vi "A01423754_Ximena_Avila_Ejercicio_16_examen_11_Febrero.vi"() -> ()   [LabVIEW 2018]
panel:
  in  "stop":bool
  out "a":bool
  out "b":bool
  out "c":bool
  out "d":bool
  out "e":bool
  out "f":bool
  out "g":bool
  out "7":bool
  out "6":bool
  out "4":bool
  out "5":bool
  out "3":bool
  out "2":bool
  out "1":bool
  in  "Boolean7":bool
  in  "Boolean6":bool
  in  "Boolean5":bool
  in  "Boolean4":bool
  in  "Boolean3":bool
  in  "Boolean2":bool
  in  "Boolean1":bool
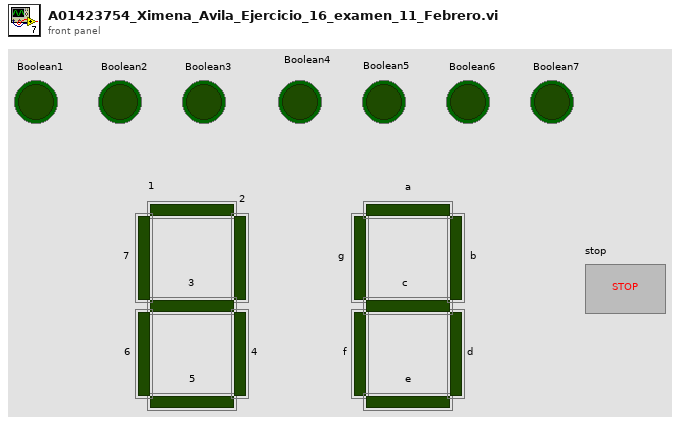
[diagram p1: front panel]
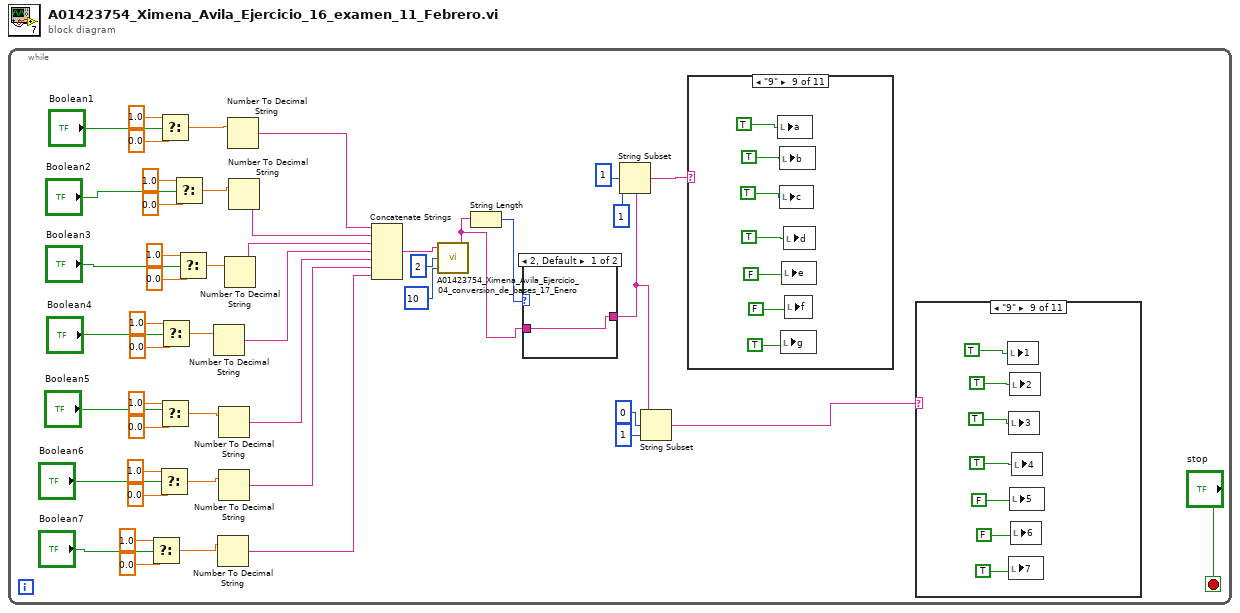
[diagram p0: block diagram]
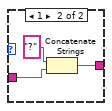
[diagram p2: hidden frame]
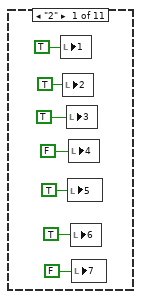
[diagram p3: hidden frame]
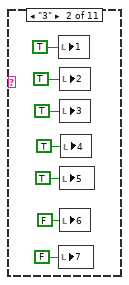
[diagram p4: hidden frame]
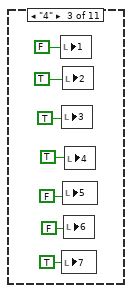
[diagram p5: hidden frame]
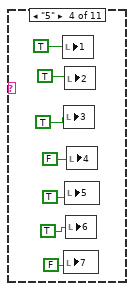
[diagram p6: hidden frame]
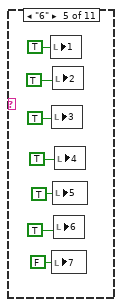
[diagram p7: hidden frame]
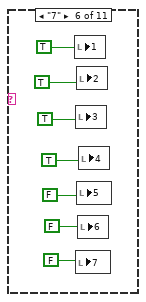
[diagram p8: hidden frame]
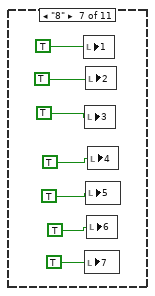
[diagram p9: hidden frame]
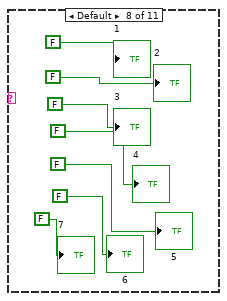
[diagram p10: hidden frame]
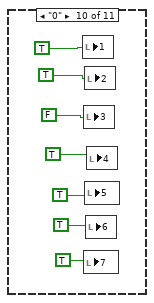
[diagram p11: hidden frame]
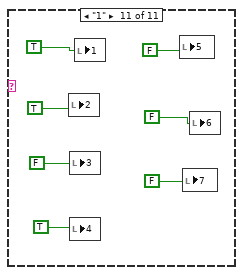
[diagram p12: hidden frame]
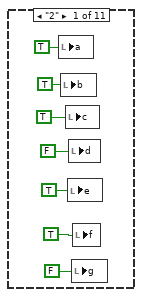
[diagram p13: hidden frame]
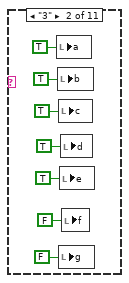
[diagram p14: hidden frame]
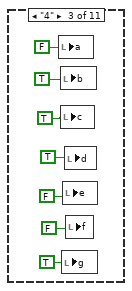
[diagram p15: hidden frame]
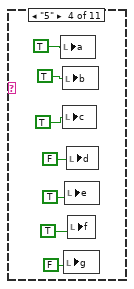
[diagram p16: hidden frame]
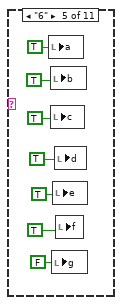
[diagram p17: hidden frame]
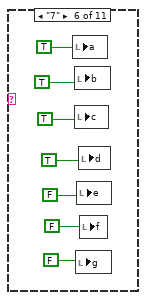
[diagram p18: hidden frame]
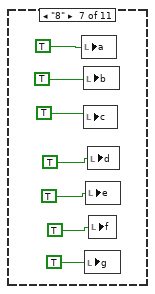
[diagram p19: hidden frame]
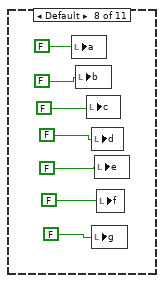
[diagram p20: hidden frame]
diagram:
  n1 = while {
    stop <- "stop" stop-if-true
    n2 = Select(t=1.0, s="Boolean7", f=0.0) -> (s? t:f=w23:dbl)
    n3 = Select(t=1.0, s="Boolean6", f=0.0) -> (s? t:f=w24:dbl)
    n4 = Select(t=1.0, s="Boolean1", f=0.0) -> (s? t:f=w29:dbl)
    n5 = Select(t=1.0, s="Boolean5", f=0.0) -> (s? t:f=w25:dbl)
    n6 = Select(t=1.0, s="Boolean4", f=0.0) -> (s? t:f=w26:dbl)
    n7 = Select(t=1.0, s="Boolean2", f=0.0) -> (s? t:f=w28:dbl)
    n8 = Select(t=1.0, s="Boolean3", f=0.0) -> (s? t:f=w27:dbl)
    n9 = Number To Decimal String(number=w26) -> (decimal integer string=w19:string)  [unwired: 1 in]
    n10 = Number To Decimal String(number=w23) -> (decimal integer string=w16:string)  [unwired: 1 in]
    n11 = Number To Decimal String(number=w25) -> (decimal integer string=w18:string)  [unwired: 1 in]
    n12 = Number To Decimal String(number=w24) -> (decimal integer string=w17:string)  [unwired: 1 in]
    n13 = Number To Decimal String(number=w27) -> (decimal integer string=w20:string)  [unwired: 1 in]
    n14 = Number To Decimal String(number=w29) -> (decimal integer string=w22:string)  [unwired: 1 in]
    n15 = Number To Decimal String(number=w28) -> (decimal integer string=w21:string)  [unwired: 1 in]
    n16 = Concatenate Strings(w22, w21, w20, w19, w18, w17, w16) -> (w15:string)
    n17 = call "A01423754_Ximena_Avila_Ejercicio_04_conversion_de_bases_17_Enero.vi"("Nueva base"=u64 10, "Base"=u64 2, "Numero"=w15) -> ("Nuevo numero"=w4:string)
    n18 = String Length(string=w4) -> (length=w5:i32)
    n19 = case shown="2, Default" w5 {
      tunnel: w4 -> [w49 w51]
      tunnel: [w49 w50] -> w3
      frame 2, Default {
      }
      frame 1 {
        n20 = Concatenate Strings("?" ("string"), w51) -> (w50:string)
      }
    }
    n21 = String Subset(string=w3, offset (0)=1, length (rest)=1 ("length (rest)")) -> (substring=w11:string)
    n22 = String Subset(string=w3, offset (0)=0, length (rest)=1 ("length (rest)")) -> (substring=w7:string)
    n23 = case shown="\"9\"" w11 {
      frame "2" {
        n24 = local write "a"(TRUE ("a")) -> ()
        n25 = local write "b"(TRUE ("b")) -> ()
        n26 = local write "c"(TRUE ("c")) -> ()
        n27 = local write "e"(TRUE ("e")) -> ()
        n28 = local write "d"(FALSE ("d")) -> ()
        n29 = local write "g"(FALSE ("g")) -> ()
        n30 = local write "f"(TRUE ("f")) -> ()
      }
      frame "3" {
        n31 = local write "a"(TRUE ("a")) -> ()
        n32 = local write "b"(TRUE ("b")) -> ()
        n33 = local write "c"(TRUE ("c")) -> ()
        n34 = local write "g"(FALSE ("g")) -> ()
        n35 = local write "e"(TRUE ("e")) -> ()
        n36 = local write "d"(TRUE ("d")) -> ()
        n37 = local write "f"(FALSE ("f")) -> ()
      }
      frame "4" {
        n38 = local write "a"(FALSE ("a")) -> ()
        n39 = local write "b"(TRUE ("a")) -> ()
        n40 = local write "c"(TRUE ("a")) -> ()
        n41 = local write "g"(TRUE ("a")) -> ()
        n42 = local write "e"(FALSE ("a")) -> ()
        n43 = local write "d"(TRUE ("a")) -> ()
        n44 = local write "f"(FALSE ("a")) -> ()
      }
      frame "5" {
        n45 = local write "a"(TRUE) -> ()
        n46 = local write "b"(TRUE) -> ()
        n47 = local write "c"(TRUE) -> ()
        n48 = local write "g"(FALSE) -> ()
        n49 = local write "e"(TRUE) -> ()
        n50 = local write "d"(FALSE) -> ()
        n51 = local write "f"(TRUE) -> ()
      }
      frame "6" {
        n52 = local write "a"(TRUE) -> ()
        n53 = local write "b"(TRUE) -> ()
        n54 = local write "c"(TRUE) -> ()
        n55 = local write "g"(FALSE) -> ()
        n56 = local write "e"(TRUE) -> ()
        n57 = local write "d"(TRUE) -> ()
        n58 = local write "f"(TRUE) -> ()
      }
      frame "7" {
        n59 = local write "a"(TRUE) -> ()
        n60 = local write "b"(TRUE) -> ()
        n61 = local write "c"(TRUE) -> ()
        n62 = local write "g"(FALSE) -> ()
        n63 = local write "e"(FALSE) -> ()
        n64 = local write "d"(TRUE) -> ()
        n65 = local write "f"(FALSE) -> ()
      }
      frame "8" {
        n66 = local write "a"(TRUE) -> ()
        n67 = local write "b"(TRUE) -> ()
        n68 = local write "c"(TRUE) -> ()
        n69 = local write "g"(TRUE) -> ()
        n70 = local write "e"(TRUE) -> ()
        n71 = local write "d"(TRUE) -> ()
        n72 = local write "f"(TRUE) -> ()
      }
      frame Default {
        n73 = local write "a"(FALSE) -> ()
        n74 = local write "b"(FALSE) -> ()
        n75 = local write "c"(FALSE) -> ()
        n76 = local write "d"(FALSE) -> ()
        n77 = local write "g"(FALSE) -> ()
        n78 = local write "e"(FALSE) -> ()
        n79 = local write "f"(FALSE) -> ()
      }
      frame "9" {
        n80 = local write "a"(TRUE) -> ()
        n81 = local write "b"(TRUE) -> ()
        n82 = local write "c"(TRUE) -> ()
        n83 = local write "g"(TRUE) -> ()
        n84 = local write "e"(FALSE) -> ()
        n85 = local write "d"(TRUE) -> ()
        n86 = local write "f"(FALSE) -> ()
      }
      frame "0" {
        n87 = local write "a"(TRUE) -> ()
        n88 = local write "b"(TRUE) -> ()
        n89 = local write "c"(FALSE) -> ()
        n90 = local write "g"(TRUE) -> ()
        n91 = local write "e"(TRUE) -> ()
        n92 = local write "d"(TRUE) -> ()
        n93 = local write "f"(TRUE) -> ()
      }
      frame "1" {
        "a" <- TRUE ("a")
        "b" <- TRUE ("b")
        "c" <- FALSE ("c")
        "d" <- TRUE ("d")
        "e" <- FALSE ("e")
        "f" <- FALSE ("f")
        "g" <- FALSE ("g")
      }
    }
    n94 = case shown="\"9\"" w7 {
      frame "2" {
        n95 = local write "1"(TRUE ("a")) -> ()
        n96 = local write "2"(TRUE ("b")) -> ()
        n97 = local write "3"(TRUE ("c")) -> ()
        n98 = local write "5"(TRUE ("e")) -> ()
        n99 = local write "4"(FALSE ("d")) -> ()
        n100 = local write "6"(TRUE ("f")) -> ()
        n101 = local write "7"(FALSE ("g")) -> ()
      }
      frame "3" {
        n102 = local write "1"(TRUE ("a")) -> ()
        n103 = local write "7"(FALSE ("g")) -> ()
        n104 = local write "2"(TRUE ("b")) -> ()
        n105 = local write "3"(TRUE ("c")) -> ()
        n106 = local write "5"(TRUE ("e")) -> ()
        n107 = local write "6"(FALSE ("f")) -> ()
        n108 = local write "4"(TRUE ("d")) -> ()
      }
      frame "4" {
        n109 = local write "1"(FALSE ("a")) -> ()
        n110 = local write "3"(TRUE ("a")) -> ()
        n111 = local write "7"(TRUE ("a")) -> ()
        n112 = local write "2"(TRUE ("a")) -> ()
        n113 = local write "5"(FALSE ("a")) -> ()
        n114 = local write "6"(FALSE ("a")) -> ()
        n115 = local write "4"(TRUE ("a")) -> ()
      }
      frame "5" {
        n116 = local write "1"(TRUE) -> ()
        n117 = local write "3"(TRUE) -> ()
        n118 = local write "7"(FALSE) -> ()
        n119 = local write "2"(TRUE) -> ()
        n120 = local write "5"(TRUE) -> ()
        n121 = local write "6"(TRUE) -> ()
        n122 = local write "4"(FALSE) -> ()
      }
      frame "6" {
        n123 = local write "1"(TRUE) -> ()
        n124 = local write "3"(TRUE) -> ()
        n125 = local write "7"(FALSE) -> ()
        n126 = local write "2"(TRUE) -> ()
        n127 = local write "5"(TRUE) -> ()
        n128 = local write "6"(TRUE) -> ()
        n129 = local write "4"(TRUE) -> ()
      }
      frame "7" {
        n130 = local write "1"(TRUE) -> ()
        n131 = local write "3"(TRUE) -> ()
        n132 = local write "7"(FALSE) -> ()
        n133 = local write "2"(TRUE) -> ()
        n134 = local write "5"(FALSE) -> ()
        n135 = local write "6"(FALSE) -> ()
        n136 = local write "4"(TRUE) -> ()
      }
      frame "8" {
        n137 = local write "1"(TRUE) -> ()
        n138 = local write "3"(TRUE) -> ()
        n139 = local write "7"(TRUE) -> ()
        n140 = local write "2"(TRUE) -> ()
        n141 = local write "5"(TRUE) -> ()
        n142 = local write "6"(TRUE) -> ()
        n143 = local write "4"(TRUE) -> ()
      }
      frame Default {
        "1" <- FALSE
        "2" <- FALSE
        "3" <- FALSE
        "4" <- FALSE
        "5" <- FALSE
        "6" <- FALSE
        "7" <- FALSE
      }
      frame "9" {
        n144 = local write "1"(TRUE) -> ()
        n145 = local write "3"(TRUE) -> ()
        n146 = local write "7"(TRUE) -> ()
        n147 = local write "2"(TRUE) -> ()
        n148 = local write "5"(FALSE) -> ()
        n149 = local write "6"(FALSE) -> ()
        n150 = local write "4"(TRUE) -> ()
      }
      frame "0" {
        n151 = local write "1"(TRUE) -> ()
        n152 = local write "3"(FALSE) -> ()
        n153 = local write "7"(TRUE) -> ()
        n154 = local write "2"(TRUE) -> ()
        n155 = local write "5"(TRUE) -> ()
        n156 = local write "6"(TRUE) -> ()
        n157 = local write "4"(TRUE) -> ()
      }
      frame "1" {
        n158 = local write "2"(TRUE ("b")) -> ()
        n159 = local write "3"(FALSE ("c")) -> ()
        n160 = local write "4"(TRUE ("d")) -> ()
        n161 = local write "1"(TRUE ("a")) -> ()
        n162 = local write "5"(FALSE ("e")) -> ()
        n163 = local write "7"(FALSE ("g")) -> ()
        n164 = local write "6"(FALSE ("f")) -> ()
      }
    }
  }
